vi "createFileStrucChop.vi"(6 "i_iter":i32, 7 "i_delay":i32, 9 "meas_path":path) -> (0 "AVG file off":path, 1 "AVG file on":path, 2 "RAW file off":path, 3 "RAW file on":path)   [LabVIEW 2015]
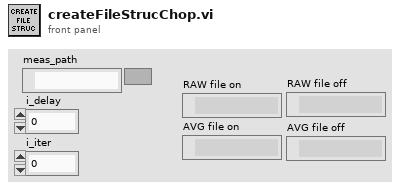
[diagram p1: front panel]
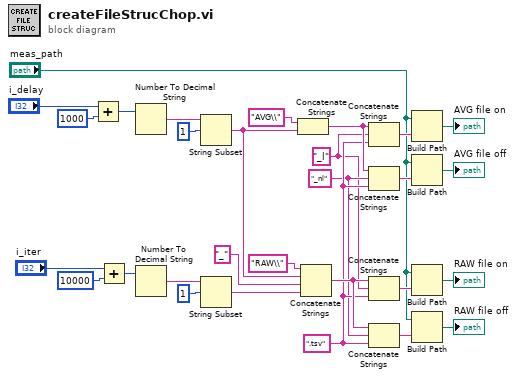
[diagram p0: block diagram]
diagram:
  w4 = "_nl"
  w3 = "_l"
  w5 = ".tsv" ("string")
  n1 = Add(x="i_delay", y=1000) -> (x+y=w23:i32)
  n2 = Add(x="i_iter", y=10000) -> (x+y=w18:i32)
  n3 = Number To Decimal String(number=w23) -> (decimal integer string=w24:string)  [unwired: 1 in]
  n4 = Number To Decimal String(number=w18) -> (decimal integer string=w19:string)  [unwired: 1 in]
  n5 = String Subset(string=w24, offset (0)=1) -> (substring=w29:string)  [unwired: 1 in]
  n6 = String Subset(string=w19, offset (0)=1) -> (substring=w14:string)  [unwired: 1 in]
  n7 = Concatenate Strings("AVG\\" ("string"), w29) -> (w6:string)
  n8 = Concatenate Strings("RAW\\" ("string"), w29, "_" ("string"), w14) -> (w12:string)
  n9 = Concatenate Strings(w6, w3, w5) -> (w8:string)
  n10 = Concatenate Strings(w6, w4, w5) -> (w9:string)
  n11 = Concatenate Strings(w12, w3, w5) -> (w13:string)
  n12 = Concatenate Strings(w12, w4, w5) -> (w10:string)
  n13 = Build Path(base path="meas_path", name or relative path=w8) -> (appended path=→"AVG file on":path)
  n14 = Build Path(base path="meas_path", name or relative path=w9) -> (appended path=→"AVG file off":path)
  n15 = Build Path(base path="meas_path", name or relative path=w13) -> (appended path=→"RAW file on":path)
  n16 = Build Path(base path="meas_path", name or relative path=w10) -> (appended path=→"RAW file off":path)
